vi "ADIS16448 Loop Update Globals.vi"(8 "error in (no error)":errorcluster, 10 "Data In":dbl[](array[numeric])) -> (0 "error out":errorcluster)   [LabVIEW 2019]
uses:
  ADIS16448 Globals.vi
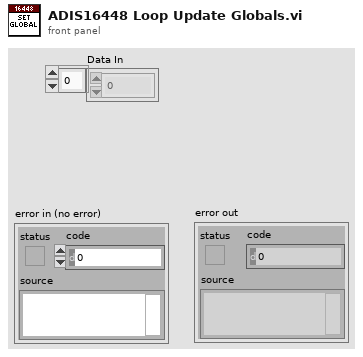
[diagram p1: front panel]
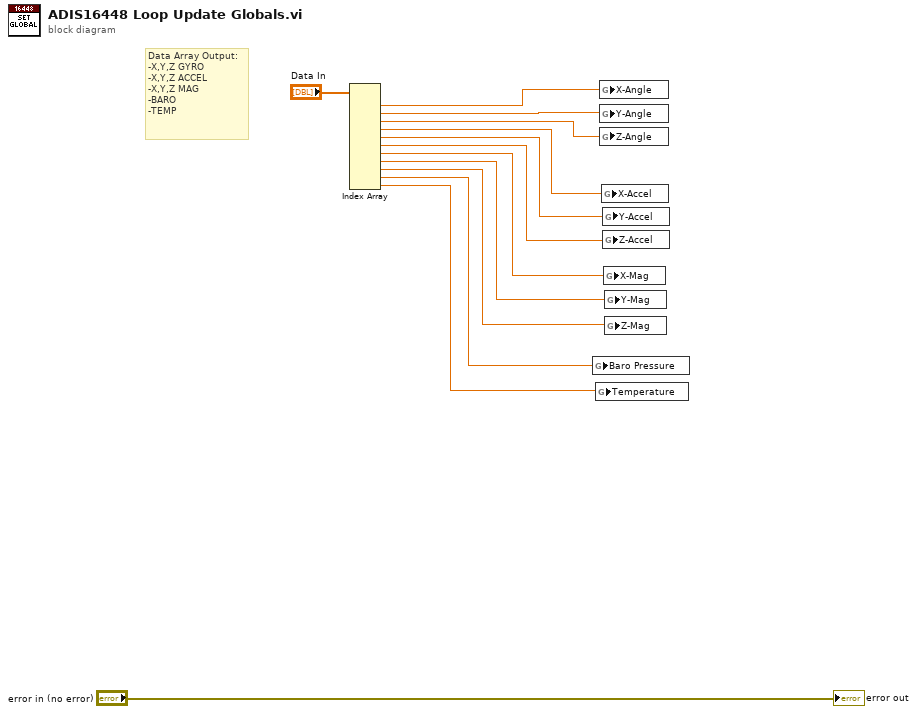
[diagram p0: block diagram]
diagram:
  # "Data Array Output:\n-X,Y,Z GYRO\n-X,Y,Z ACCEL\n-X,Y,Z MAG\n-BARO\n-TEMP"
  n1 = Index Array(array="Data In") -> (element #1=w12:dbl, element #2=w11:dbl, element #3=w10:dbl, element #4=w9:dbl, element #5=w8:dbl, element #6=w7:dbl, element #7=w6:dbl, element #8=w5:dbl, element #9=w4:dbl, element #10=w3:dbl, element #11=w2:dbl)  [unwired: 11 in]
  n2 = global write "ADIS16448 Globals.vi" "Baro Pressure"(w3) -> ()
  n3 = global write "ADIS16448 Globals.vi" "Temperature"(w2) -> ()
  n4 = global write "ADIS16448 Globals.vi" "X-Angle"(w12) -> ()
  n5 = global write "ADIS16448 Globals.vi" "Y-Angle"(w11) -> ()
  n6 = global write "ADIS16448 Globals.vi" "Z-Angle"(w10) -> ()
  n7 = global write "ADIS16448 Globals.vi" "X-Accel"(w9) -> ()
  n8 = global write "ADIS16448 Globals.vi" "Y-Accel"(w8) -> ()
  n9 = global write "ADIS16448 Globals.vi" "Z-Accel"(w7) -> ()
  n10 = global write "ADIS16448 Globals.vi" "X-Mag"(w6) -> ()
  n11 = global write "ADIS16448 Globals.vi" "Y-Mag"(w5) -> ()
  n12 = global write "ADIS16448 Globals.vi" "Z-Mag"(w4) -> ()
  "error out" <- "error in (no error)"
